vi "CTRE_PigeonIMU_GetAccumGyro.vi"(8 "error in (no error)":errorcluster, 11 "PigeonIMUDevRef":T1={"DeviceStatus"={"status"=FALSE, "code"=0, "source"=""}, "Device Number"=0, "Type"=352321536, "Device ID"=0, "Handle"=0, "UsageFrame"=0, "Library Path"=path ""} {"Type" items=["CAN"=352321536, "TalonSRX"=33554432]}) -> (0 "error out":errorcluster, 2 "AccumGyro":cluster{"X":dbl, "Y":dbl, "Z":dbl}, 3 "PigeonIMUDevRef":T1={"DeviceStatus"={"status"=FALSE, "code"=0, "source"=""}, "Device Number"=0, "Type"=352321536, "Device ID"=0, "Handle"=0, "UsageFrame"=0, "Library Path"=path ""} {"Type" items=["CAN"=352321536, "TalonSRX"=33554432]})   [LabVIEW 2016]
uses:
  <vilib>/Rock Robotics/WPI/ThirdParty/Sensors/Pigeon IMU/CTRE_PigeonIMU_DeviceRef.ctl
  <vilib>/Rock Robotics/WPI/ThirdParty/Sensors/Pigeon IMU/CTRE_PigeonIMU_ConnectionType.ctl
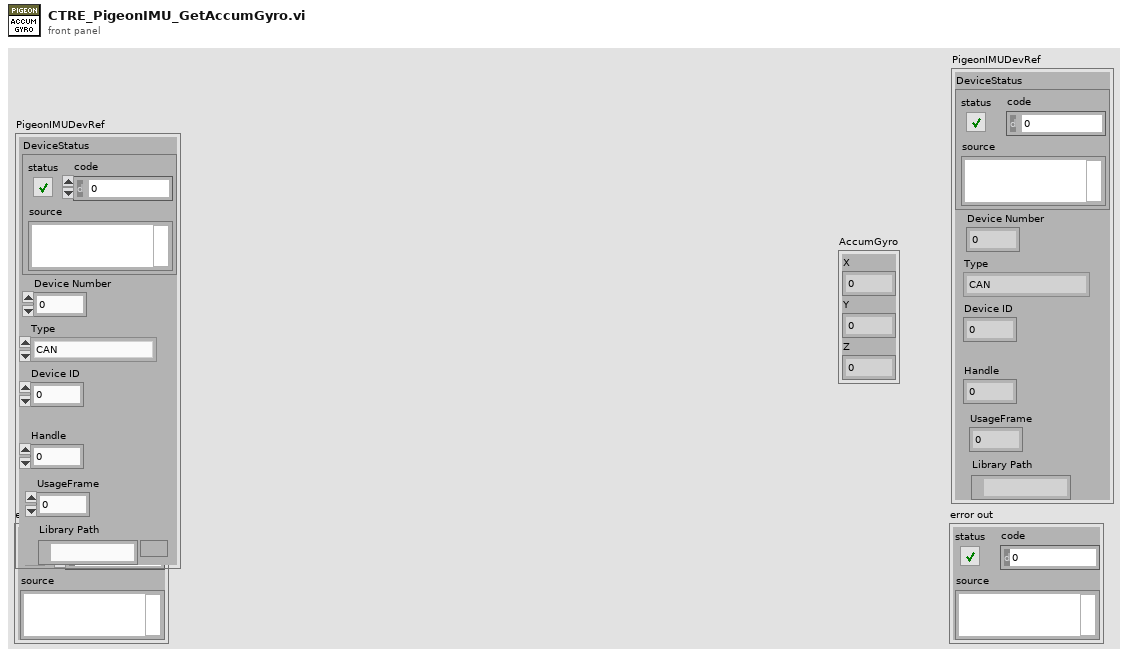
[diagram p1: front panel]
types:
  T1 = typedef "CTRE_PigeonIMU_DeviceRef.ctl" = cluster{"DeviceStatus":errorcluster, "Device Number":u8, "Type":T2, "Device ID":u32, "Handle":u64, "UsageFrame":u32, "Library Path":path}
  T2 = typedef "CTRE_PigeonIMU_ConnectionType.ctl" = u32
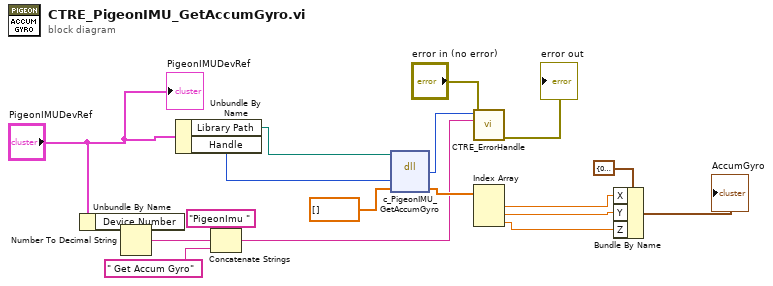
[diagram p0: block diagram]
diagram:
  n1 = Unbundle By Name("PigeonIMUDevRef") -> ("Device Number"=w9:u8)
  n2 = Number To Decimal String(number=w9) -> (decimal integer string=w8:string)  [unwired: 1 in]
  n3 = Unbundle By Name("PigeonIMUDevRef") -> ("Library Path"=w18:path, "Handle"=w17:u64)
  n4 = Concatenate Strings("PigeonImu " ("string"), w8, " Get Accum Gyro" ("string")) -> (w2:string)
  n5 = dll-call lib="?" fn="c_PigeonIMU_GetAccumGyro"(path in=w18, "handle"=w17, "xyz_deg"=dbl[] []) -> ("return type"=w1:i32, "xyz_deg"=w15:dbl[])  [unwired: 3 in, 2 out]
  n6 = call <vilib>:"CTRE_ErrorHandle.vi"("error in"="error in (no error)", "origin"=w2, "code"=w1) -> ("error out"=→"error out":errorcluster)  [unwired: 8 in]
  n7 = Index Array(array=w15) -> (element #1=w12:dbl, element #2=w11:dbl, element #3=w10:dbl)  [unwired: 3 in]
  n8 = Bundle By Name(cluster=cluster{"X":dbl, "Y":dbl, "Z":dbl} {"X"=0.0, "Y"=0.0, "Z"=0.0} ("AccumGyro"), "X"=w12, "Y"=w11, "Z"=w10) -> (→"AccumGyro":cluster{"X":dbl, "Y":dbl, "Z":dbl})
  "PigeonIMUDevRef" <- "PigeonIMUDevRef"
